vi "VI Tree.vi"   [LabVIEW 2012, in "Phidget Spatial.lvlib"]
doc: "${Spatial:VITreeHeader}"
uses:
  <instrlib>/Phidgets/Phidget Spatial/Phidget Spatial.lvlib
  <instrlib>/Phidgets/Phidget Spatial/Public/SpatialStart.vi
  <instrlib>/Phidgets/Phidget Spatial/Public/SpatialOpen.vi
  <instrlib>/Phidgets/Phidget Spatial/Public/SpatialClose.vi
panel:
  # "(c) 2015 Phidgets Inc..  ALL RIGHTS RESERVED."
  # "SEE DIAGRAM\nFOR VI TREE."
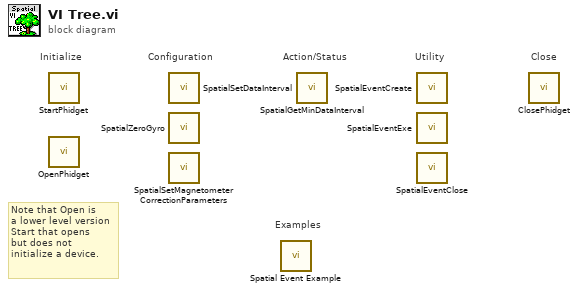
[diagram p0: block diagram]
diagram:
  # "Note that Open is\na lower level version\nStart that opens\nbut does not \ninitialize a device."
  # "Examples"
  # "Configuration"
  # "Utility"
  # "Action/Status"
  # "Close"
  # "Initialize"
  n1 = call-poly <instrlib>:"StartPhidget.vi"() -> ()  [unwired: 12 in, 4 out]
  n2 = call-poly <instrlib>:"OpenPhidget.vi"() -> ()  [unwired: 8 in, 4 out]
  n3 = call <instrlib>:"SpatialSetDataInterval.vi"() -> ()  [unwired: 9 in, 2 out]
  n4 = call <instrlib>:"SpatialZeroGyro.vi"() -> ()  [unwired: 9 in, 2 out]
  n5 = call <instrlib>:"SpatialSetMagnetometerCorrectionParameters.vi"() -> ()  [unwired: 9 in, 2 out]
  n6 = call <instrlib>:"Spatial Event Example.vi"() -> ()  [unwired: 12 in]
  n7 = call <instrlib>:"SpatialGetMinDataInterval.vi"() -> ()  [unwired: 8 in, 3 out]
  n8 = call <instrlib>:"SpatialEventCreate.vi"() -> ()  [unwired: 9 in, 3 out]
  n9 = call <instrlib>:"SpatialEventExe.vi"() -> ()  [unwired: 18 in, 10 out]
  n10 = call <instrlib>:"SpatialEventClose.vi"() -> ()  [unwired: 10 in, 2 out]
  n11 = call-poly <instrlib>:"ClosePhidget.vi"() -> ()  [unwired: 11 in, 1 out]
